vi "Get Port Simulated.vi"(10 "Buttons":bool[](array[boolean]), 11 "Exprected Response":string) -> (2 "Port":string, 3 "Response":string)   [LabVIEW 2020, in "UI Actor.lvlib" / "UI Actor.lvclass"]
uses:
  UI Actor.lvclass
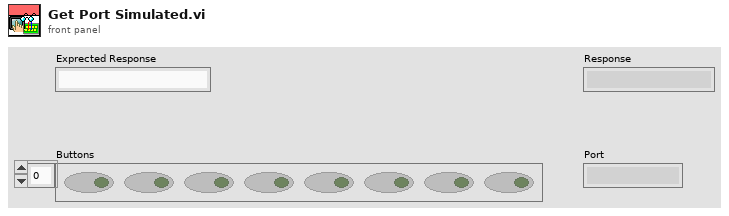
[diagram p1: front panel]
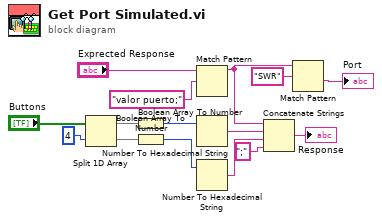
[diagram p0: block diagram]
diagram:
  n1 = Split 1D Array(array="Buttons", index=4) -> (first subarray=w12:bool[], second subarray=w11:bool[])
  n2 = Boolean Array To Number(Boolean array=w12) -> (number=w9:u32)
  n3 = Boolean Array To Number(Boolean array=w11) -> (number=w10:u32)
  n4 = Match Pattern(string="Exprected Response", regular expression="valor puerto;") -> (before substring=w3:string)  [unwired: 1 in, 3 out]
  n5 = Number To Hexadecimal String(2:w9) -> (0:w6:string)  [unwired: 1 in]
  n6 = Number To Hexadecimal String(2:w10) -> (0:w5:string)  [unwired: 1 in]
  n7 = Concatenate Strings(w3, w6, w5, ";" ("string")) -> (→"Response":string)
  n8 = Match Pattern(string=w3, regular expression="SWR") -> (after substring=→"Port":string)  [unwired: 1 in, 3 out]
